vi "Test Eng Database.vi"() -> ()   [LabVIEW 2021]
uses:
  <vilib>/addons/database/Auxilliary.llb/DB Tools Cursor Type.ctl
  <vilib>/addons/database/Connection.llb/DB Tools Open Connec (Path).vi
  <vilib>/addons/database/Connection.llb/Conn Execute.vi
  <vilib>/addons/database/Recordset.llb/Rec Fetch Recordset Data (R).vi
  <vilib>/addons/database/_DB Variant To Data/Database Variant To Data.xnode
  <vilib>/addons/database/NI_Database_API.lvlib
panel:
  in  "error in (no error)":errorcluster
  out "error out":errorcluster
  in  "ShowAll":bool
  out "SQL Query":string
  in  "New":bool
  in  "Eq ID":string
  out "DataList":i32(listbox)
  in  "Salir":bool
  in  "Search":bool
  in  "Keyword":string
  # "Search"
  # "Corrective Maintenance \nTroubleshooting Log"
  # "Keyword:"
  # "Equipment ID:"
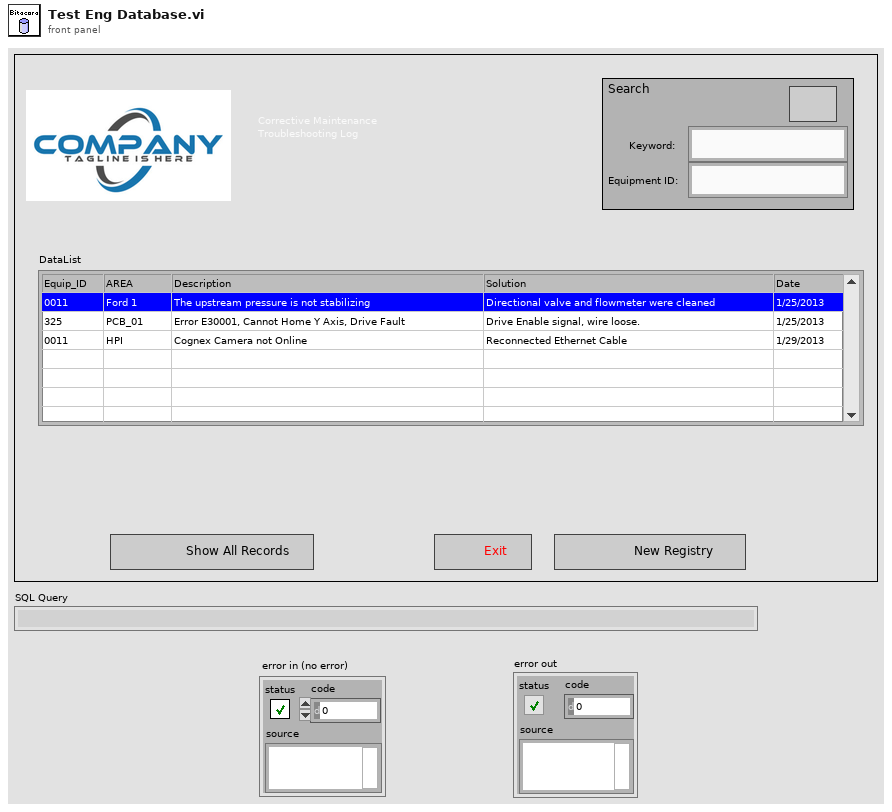
[diagram p1: front panel]
types:
  T1 = typedef "NI_Database_API.lvlib/Conn ObjectReference.ctl" = refnum<k1>
  T2 = typedef "NI_Database_API.lvlib/DB Tools Cursor Type.ctl" = enum16{"forward-only", "keyset", "dynamic", "static"}
  T3 = typedef "NI_Database_API.lvlib/Rec ObjectReference.ctl" = refnum<k1>
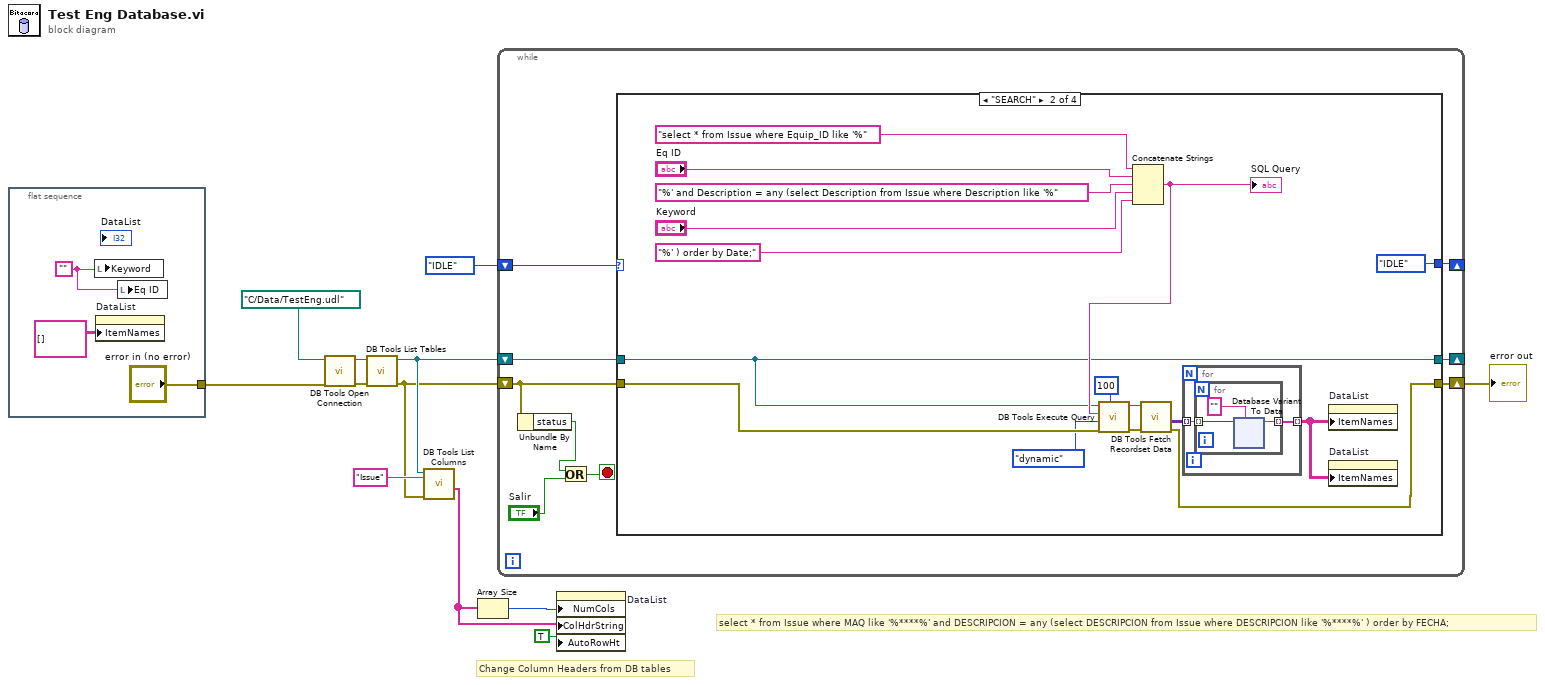
[diagram p0: block diagram]
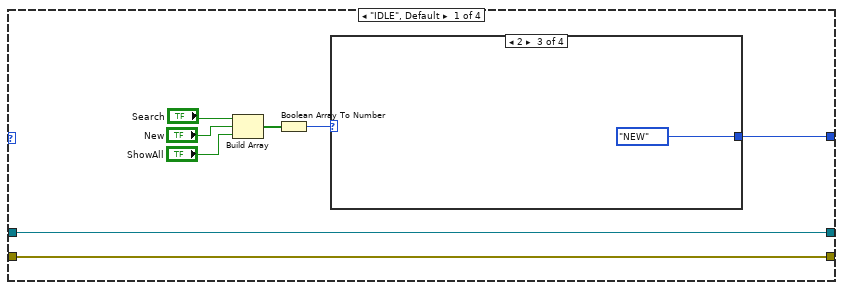
[diagram p2: hidden frame]
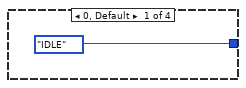
[diagram p3: hidden frame]
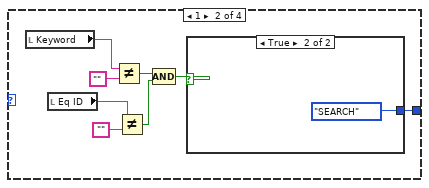
[diagram p4: hidden frame]
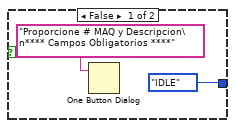
[diagram p5: hidden frame]
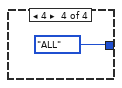
[diagram p6: hidden frame]
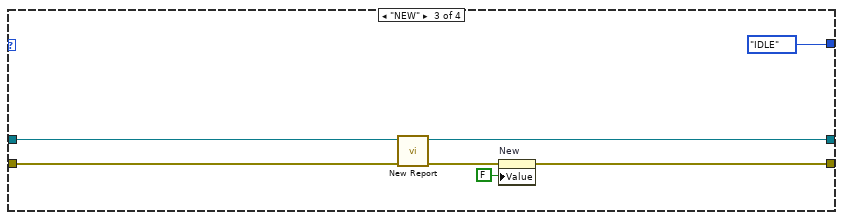
[diagram p7: hidden frame]
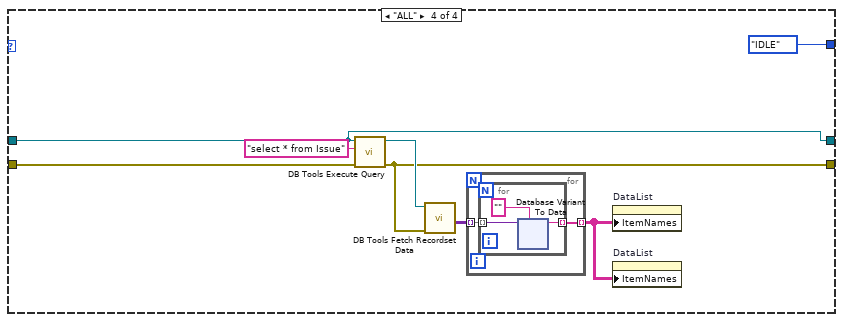
[diagram p8: hidden frame]
diagram:
  # "Change Column Headers from DB tables"
  # "select * from Issue where MAQ like '%****%' and DESCRIPCION = any (select DESCRIPCION from Issue where DESCRIPCION like '%****%' ) order by FECHA;"
  n1 = flat-sequence {
    tunnel: ["error in (no error)"] -> w1
    frame #0 {
      w15 = ""
      n2 = local write "Keyword"(w15) -> ()
      n3 = property on="DataList" class="MCListbox (strict)"("ItemNames"=string[][] [] ("Item Names")) -> ()  [unwired: 2 in, 2 out]
      n4 = local write "Eq ID"(w15) -> ()
    }
  }
  n5 = call-poly <vilib>:"DB Tools Open Connection.vi"("error in (no error)"=w1, "connection information"=path "C:/Data/TestEng.udl" ("Application:Directory Path")) -> ("error out"=w12:errorcluster, "connection reference"=w11:T1)  [unwired: 6 in]
  n6 = call <vilib>:"DB Tools List Tables.vi"("error in (no error)"=w12, "connection reference"=w11) -> ("error out"=w3:errorcluster, "connection reference out"=w6:T1)  [unwired: 3 in, 1 out]
  n7 = call <vilib>:"DB Tools List Columns.vi"("error in (no error)"=w3, "table"="Issue", "connection reference"=w6) -> ("columns"=w4:string[])  [unwired: 1 in, 3 out]
  n8 = Array Size(array=w4) -> (size(s)=w8:i32)
  n9 = while {
    shift-right: [w23] -> _
    shift-left: w6 -> [w24]
    shift-right: [w21] -> _
    shift-left: enum16{"IDLE", "SEARCH", "NEW", "ALL"}."IDLE" -> [w22]
    shift-right: [w20] -> w2
    shift-left: w3 -> [w19]
    stop <- w16 stop-if-true
    n10 = Unbundle By Name(w19) -> ("status"=w18:bool)
    n11 = Or(x=w18, y="Salir") -> (x .or. y?=w16:bool)
    n12 = case shown="\"SEARCH\"" w22 {
      tunnel: w24 -> [w32 w49 w106 w108]
      tunnel: [w32 w49 w105 w108] -> w23
      tunnel: [w28 enum16{"IDLE", "SEARCH", "NEW", "ALL"}."IDLE" enum16{"IDLE", "SEARCH", "NEW"}."IDLE" enum16{"IDLE", "SEARCH", "NEW", "ALL"}."IDLE"] -> w21
      tunnel: w19 -> [w26 w56 w104 w111]
      tunnel: [w26 w55 w102 w107] -> w20
      frame "IDLE", Default {
        n13 = Build Array("Search", "New", "ShowAll") -> (w30:bool[])
        n14 = Boolean Array To Number(Boolean array=w30) -> (number=w29:u32)
        n15 = case shown="2" w29 {
          tunnel: [enum16{"IDLE", "SEARCH"}."IDLE" w34 enum16{"IDLE", "SEARCH", "NEW"}."NEW" enum16{"IDLE", "SEARCH", "NEW", "ALL"}."ALL"] -> w28
          frame 0, Default {
          }
          frame 1 {
            n16 = local read "Keyword"() -> (w37:string)
            n17 = local read "Eq ID"() -> (w39:string)
            n18 = Not Equal?(x=w37, y="") -> (x != y?=w40:bool)
            n19 = Not Equal?(x=w39, y="") -> (x != y?=w41:bool)
            n20 = Compound Arithmetic op=AND(w40, w41) -> (w35:bool)
            n21 = case shown="True" w35 {
              tunnel: [enum16{"IDLE", "SEARCH"}."IDLE" enum16{"IDLE", "SEARCH"}."SEARCH"] -> w34
              frame False {
                n22 = One Button Dialog(message="Proporcione # MAQ y Descripcion\n**** Campos Obligatorios ****" ("table")) -> ()  [unwired: 1 in, 1 out]
              }
              frame True {
              }
            }
          }
          frame 2 {
          }
          frame 4 {
          }
        }
      }
      frame "SEARCH" {
        n23 = Concatenate Strings("select * from Issue where Equip_ID like '%", "Eq ID", "%' and Description = any (select Description from Issue where Description like '%" ("string"), "Keyword", "%' ) order by Date;") -> (w52:string)
        "SQL Query" <- w52
        n24 = call-poly <vilib>:"DB Tools Execute Query.vi"("cache size (1)"=100, "error in (no error)"=w56, "cursor type"=DB_Tools_Cursor_Type."dynamic", "SQL query"=w52, "connection reference"=w49) -> ("error out"=w62:errorcluster, "recordset reference"=w61:T3)  [unwired: 3 in]
        n25 = call-poly <vilib>:"DB Tools Fetch Recordset Data.vi"("error in (no error)"=w62, "recordset reference"=w61) -> ("error out"=w55:errorcluster, "recordset data"=w47:variant[][])  [unwired: 3 in, 1 out]
        n26 = for {
          tunnel: [w64] -> w59 mode=indexing
          tunnel: w47 -> [w63] mode=indexing
          n27 = for {
            tunnel: [w67] -> w64 mode=indexing
            tunnel: w63 -> [w65] mode=indexing
            n28 = xnode "Database Variant To Data"("database variant"=w65, "type"="") -> ("data"=w67:string)  [unwired: 1 in, 1 out]
          }
        }
        n29 = property on="DataList" class="MCListbox (strict)"("ItemNames"=w59) -> ()  [unwired: 2 in, 2 out]
        n30 = property on="DataList" class="MCListbox (strict)"("ItemNames"=w59) -> ()  [unwired: 2 in, 2 out]
      }
      frame "NEW" {
        n31 = call "New Report.vi"("error in"=w104, "connection reference"=w106) -> ("error out"=w103:errorcluster, "connection reference 2"=w105:T1)  [unwired: 8 in]
        n32 = property on="New" class="Bool (strict)"(error in=w103, "Value"=FALSE ("Crear Nuevo")) -> (error out=w102:errorcluster)  [unwired: 1 in, 1 out]
      }
      frame "ALL" {
        n33 = call-poly <vilib>:"DB Tools Execute Query.vi"("error in (no error)"=w111, "SQL query"="select * from Issue", "connection reference"=w108) -> ("error out"=w107:errorcluster, "recordset reference"=w114:T3)  [unwired: 5 in]
        n34 = call-poly <vilib>:"DB Tools Fetch Recordset Data.vi"("error in (no error)"=w107, "recordset reference"=w114) -> ("recordset data"=w113:variant[][])  [unwired: 3 in, 2 out]
        n35 = for {
          tunnel: w113 -> [w116] mode=indexing
          tunnel: [w115] -> w112 mode=indexing
          n36 = for {
            tunnel: w116 -> [w119] mode=indexing
            tunnel: [w118] -> w115 mode=indexing
            n37 = xnode "Database Variant To Data"("database variant"=w119, "type"="") -> ("data"=w118:string)  [unwired: 1 in, 1 out]
          }
        }
        n38 = property on="DataList" class="MCListbox (strict)"("ItemNames"=w112) -> ()  [unwired: 2 in, 2 out]
        n39 = property on="DataList" class="MCListbox (strict)"("ItemNames"=w112) -> ()  [unwired: 2 in, 2 out]
      }
    }
  }
  "error out" <- w2
  n40 = property on="DataList" class="MCListbox (strict)"("NumCols"=w8, "ColHdrString"=w4, "AutoRowHt"=TRUE ("Autosizing Row Height")) -> ()  [unwired: 2 in, 2 out]
